vi "Kelvinox_Parse_Heater_Number_to_Excitation.vi"(1 "Excitation Level":dbl) -> (0 "Excitation String":string)   [LabVIEW 2019]
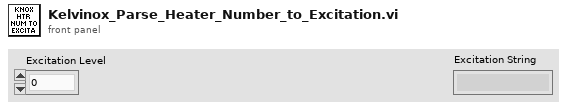
[diagram p1: front panel]
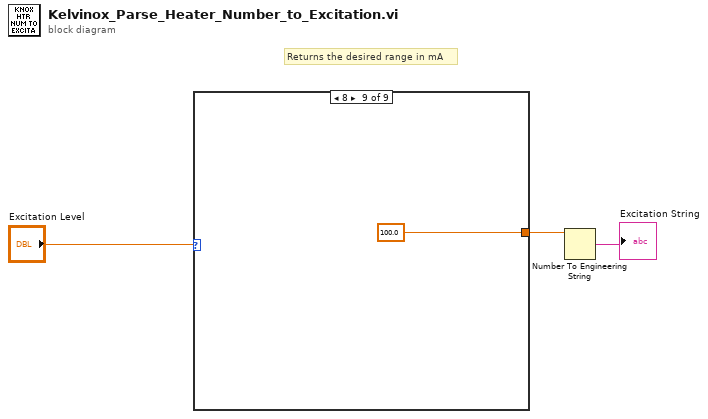
[diagram p0: block diagram]
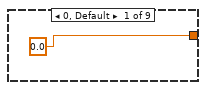
[diagram p2: hidden frame]
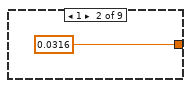
[diagram p3: hidden frame]
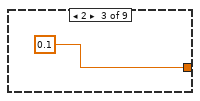
[diagram p4: hidden frame]
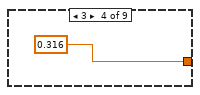
[diagram p5: hidden frame]
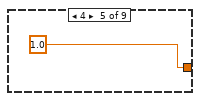
[diagram p6: hidden frame]
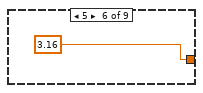
[diagram p7: hidden frame]
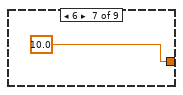
[diagram p8: hidden frame]
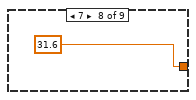
[diagram p9: hidden frame]
diagram:
  # "Returns the desired range in mA"
  n1 = case shown="8" "Excitation Level" {
    tunnel: [0.0 0.0316 0.1 0.316 1.0 3.16 10.0 31.6 100.0] -> w1
    frame 0, Default {
    }
    frame 1 {
    }
    frame 2 {
    }
    frame 3 {
    }
    frame 4 {
    }
    frame 5 {
    }
    frame 6 {
    }
    frame 7 {
    }
    frame 8 {
    }
  }
  n2 = Number To Engineering String(4:w1) -> (0:→"Excitation String":string)  [unwired: 3 in]
